vi "Ximea Set ROI.vi"(8 "error in":errorcluster, 9 "Image Ref":T6, 10 "Ximea Camera Cluster":T1, 11 "xiCam In":refnum<k24>) -> (0 "error out":errorcluster, 3 "xiCam Out":refnum<k24>)   [LabVIEW 2016]
uses:
  C:/Users/Ries Lab/Documents/Microscope Control from Sheng Account/Microscope-Control/Device Library/Cameras/Ximea/xiLIB_64bit/xiLIB/xiCamLib/API/x64/xiApi.NETX64.dll
  xiLIB_64bit/xiLIB/xiCamLib/API/x64/xiApi.NETX64.dll
  <vilib>/vision/Image Controls.llb/IMAQ Image.ctl
  Ximea Controls/Ximea Notifier Element.ctl
  Ximea Controls/Ximea Actions.ctl
  Ximea Controls/Ximea Parameters.ctl
  Ximea Controls/Ximea Parameter List.ctl
  Ximea Controls/Ximea ROI.ctl
  Camera Controls/Camera IMAQ Key Info.ctl
  xiLIB_64bit/xiLIB/xiCamLib/xiCam/PRM/PRM/PRM_v2.ctl
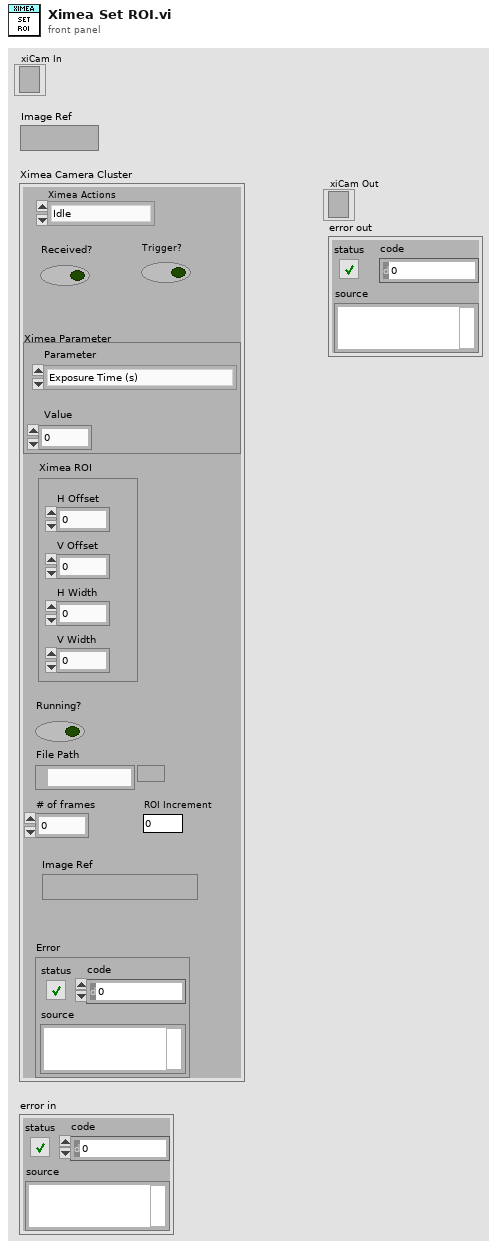
[diagram p1: front panel]
types:
  T1 = typedef "Ximea Notifier Element.ctl" = cluster{"Ximea Actions":T2, "Received?":bool, "Ximea Parameter":T3, "Ximea ROI":T5, "Running?":bool, "File Path":path, "# of frames":u32, "Image Ref":T6, "Error":errorcluster, "Trigger?":bool, "ROI Increment":i32}
  T2 = typedef "Ximea Actions.ctl" = enum16{"Idle", "Error Check", "Preview", "Record", "Soft Trigger", "Abort", "Record Settings", "Set Parameter", "Get Parameter", "Set ROI", "Get ROI", "Status", "Quit"}
  T3 = typedef "Ximea Parameters.ctl" = cluster{"Parameter":T4, "Value":sgl}
  T4 = typedef "Ximea Parameter List.ctl" = enum16{"Exposure Time (s)", "Gain"}
  T5 = typedef "Ximea ROI.ctl" = cluster{"H Offset":i32, "V Offset":i32, "H Width":i32, "V Width":i32}
  T6 = typedef "IMAQ Image.ctl" = refnum<image>
  T7 = typedef "PRM_v2.ctl" = enum16{"ACQ_BUFFER_SIZE", "ACQ_FRAME_BURST_COUNT", "ACQ_TIMING_MODE", "ACQ_TRANSPORT_BUFFER_SIZE", "AE_MAX_LIMIT", "AEAG", "AEAG_LEVEL", "API_VERSION", "AG_MAX_LIMIT", "APPLY_CMS", "AUTO_BANDWIDTH_CALCULATION", "AUTO_WB", "AVAILABLE_BANDWIDTH", "AVAILABLE_BANDWIDTH_MAX", "AVAILABLE_BANDWIDTH_MIN", "BUFFER_POLICY", "BUFFERS_QUEUE_SIZE", "CC_MATRIX_00", "CC_MATRIX_01", "CC_MATRIX_02", "CC_MATRIX_03", "CC_MATRIX_10", "CC_MATRIX_11", "CC_MATRIX_12", "CC_MATRIX_13", "CC_MATRIX_20", "CC_MATRIX_21", "CC_MATRIX_22", "CC_MATRIX_23", "CC_MATRIX_30", "CC_MATRIX_31", "CC_MATRIX_32", "CC_MATRIX_33", "CHIP_TEMP", "CMS", "COLOR_FILTER_ARRAY", "COOLING", "DEBOUNCE_EN", "DEBOUNCE_POL", "DEBOUNCE_T0", "DEBOUNCE_T1", "DEBUG_LEVEL", "DEFAULT_CC_MATRIX", "DEVICE_INSTANCE_PATH", "DEVICE_MODEL_ID", "DEVICE_NAME", "DEVICE_SN", "DEVICE_TYPE", "DEVICE_USER_ID", "DOWNSAMPLING", "DOWNSAMPLING_TYPE", "DRV_VERSION", "EXP_PRIORITY", "EXPOSURE", "EXPOSURE_MAX", "EXPOSURE_MIN", "FFS_FILE_NAME", "FPGA1_VERSION", "FRAMERATE", "FRAMERATE_MAX", "FRAMERATE_MIN", "FREE_FFS_SIZE", "GAIN", "GAIN_MAX", "GAIN_MIN", "GAMMAC", "GAMMAY", "GPI_LEVEL", "GPI_MODE", "GPI_SELECTOR", "GPO_MODE", "GPO_SELECTOR", "HDR", "HDR_T1", "HDR_T2", "HEIGHT", "HEIGHT_MAX", "HEIGHT_MIN", "HOUSE_TEMP", "IMAGE_DATA_FORMAT", "IMAGE_IS_COLOR", "INPUT_CMS_PROFILE", "IS_COOLED", "IS_DEVICE_EXIST", "KNEEPOINT1", "KNEEPOINT2", "LED_MODE", "LED_SELECTOR", "LIMIT_BANDWIDTH", "LIMIT_BANDWIDTH_MAX", "LIMIT_BANDWIDTH_MIN", "LUT_EN", "LUT_INDEX", "LUT_INDEX_MAX", "LUT_INDEX_MIN", "LUT_VALUE", "LUT_VALUE_MAX", "LUT_VALUE_MIN", "MANUAL_WB", "MCU1_VERSION", "MCU2_VERSION", "OFFSET_X", "OFFSET_X_MAX", "OFFSET_X_MIN", "OFFSET_Y", "OFFSET_Y_MAX", "OFFSET_Y_MIN", "OUTPUT_CMS_PROFILE", "OUTPUT_DATA_BIT_DEPTH", "OUTPUT_DATA_PACKING", "READ_FILE_FFS", "RECENT_FRAME", "SENSOR_DATA_BIT_DEPTH", "SENSOR_MODE", "SENSOR_TAPS", "SHARPNESS", "SHUTTER_TYPE", "TARGET_TEMP", "TRG_DELAY", "TRG_SELECTOR", "TRG_SOFTWARE", "TRG_SOURCE", "USED_FFS_SIZE", "WB_KB", "WB_KG", "WB_KR", "WIDTH", "WIDTH_MAX", "WIDTH_MIN", "WRITE_FILE_FFS", "ACQ_BUFFER_SIZE_UNIT", "ACQ_TRANSPORT_BUFFER_COMMIT", "AEAG_ROI_HEIGHT", "AEAG_ROI_OFFSET_X", "AEAG_ROU_OFFSET_Y", "AEAG_ROI_WIDTH", "API_CONTEXT_LIST", "BINNING_HORIZONTAL", "BINNING_SELECTOR", "BINNING_VERTICAL", "COLUMN_FPN_CORRECTION", "COUNTER_SELECTOR", "COUNTER_VALUE", "DECIMATION_HORIZONTAL", "DECIMATION_SELECTOR", "DECIMATION_VERTICAL", "DEVICE_ID", "DEVICE_LOCATION_PATH", "DEVICE_MANIFEST", "DEVICE_RESET", "DEVICE_SENS_SN", "EXPOSURE_BURST_COUNT", "FFS_ACCESS_KEY", "GAIN_SELECTOR", "HW_REVISION", "IMAGE_BLACK_LEVEL", "IMAGE_DATA_BIT_DEPTH", "IMAGE_DATA_FORMAT_RGB32_ALPHA", "IMAGE_PAYLOAD_SIZE", "LENS_APERTURE_VALUE", "LENS_FEATURE", "LENS_FEATURE_SELECTOR", "LENS_FOCAL_LENGTH", "LENS_FOCUS_DISTANCE", "LENS_FOCUS_MOVE", "LENS_FOCUS_MOVEMENT_VALUE", "LENS_MODE", "OUTPUT_DATA_PACKING_TYPE", "SENSOR_CLOCK_FREQ_HZ", "SENSOR_CLOCK_FREQ_INDEX", "SENSOR_FEATURE_SELECTOR", "SENSOR_FEATURE_VALUE", "SENSOR_OUTPUT_CHANNEL_COUNT", "TRANSPORT_PIXEL_FORMAT", "TS_RST_MODE", "TS_RST_SOURCE", "SENS_DEFECTS_CORR_LIST_SELECTOR", "SENS_DEFECTS_CORR", "SENS_DEFECTS_CORR_LIST_CONTENT", "DEVICE_UNIT_SELECTOR", "DEVICE_UNIT_REGISTER_SELECTOR", "DEVICE_UNIT_REGISTER_VALUE"}
  T8 = typedef "Camera IMAQ Key Info.ctl" = cluster{"Frame":u32, "Sensor Height":i32, "Sensor Width":i32, "ROI Height":i32, "ROI Width":i32, "ROI Enable?":bool, "Bit per Pixel":u8}
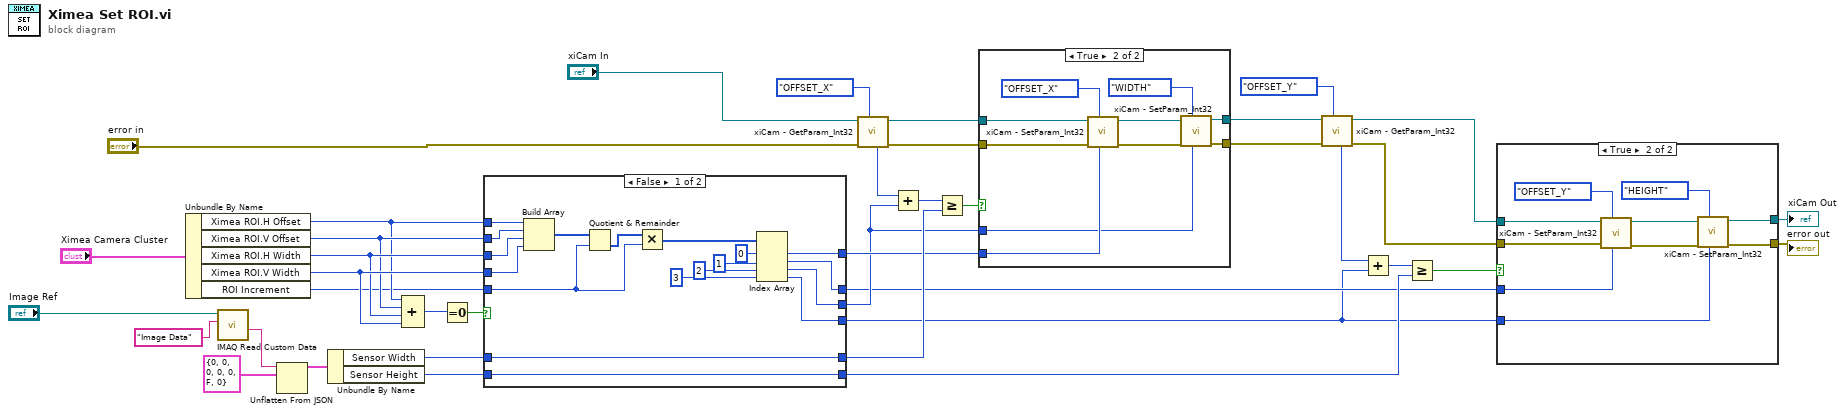
[diagram p0: block diagram]
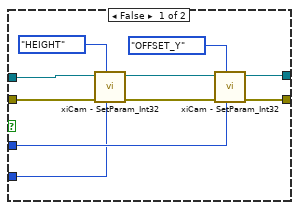
[diagram p2: hidden frame]
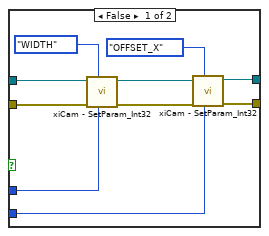
[diagram p3: hidden frame]
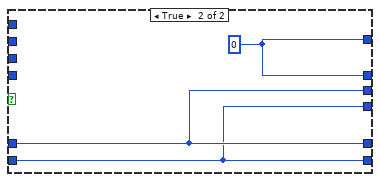
[diagram p4: hidden frame]
diagram:
  n1 = Unbundle By Name("Ximea Camera Cluster") -> ("Ximea ROI.H Offset"=w28:i32, "Ximea ROI.V Offset"=w29:i32, "Ximea ROI.H Width"=w30:i32, "Ximea ROI.V Width"=w31:i32, "ROI Increment"=w27:i32)
  n2 = call "IMAQ Read Custom Data"("Key"="Image Data", "Image"="Image Ref") -> ("Custom Data Out"=w21:string)  [unwired: 7 in, 2 out]
  n3 = Unflatten From JSON(JSON string=w21, type and defaults=T8 {"Frame"=0, "Sensor Height"=0, "Sensor Width"=0, "ROI Height"=0, "ROI Width"=0, "ROI Enable?"=FALSE, "Bit per Pixel"=0} ("Camera IMAQ Key Info")) -> (value=w22:T8)  [unwired: 5 in, 1 out]
  n4 = Unbundle By Name(w22) -> ("Sensor Width"=w25:i32, "Sensor Height"=w26:i32)
  n5 = Compound Arithmetic op=ADD(w28, w29, w30, w31) -> (w19:i32)
  n6 = Equal To 0?(x=w19) -> (x = 0?=w24:bool)
  n7 = case shown="False" w24 {
    tunnel: w25 -> [w41 w59]
    tunnel: w26 -> [w40 w58]
    tunnel: [w44 w59] -> w14
    tunnel: [w43 w58] -> w3
    tunnel: w27 -> [w48 _]
    tunnel: w28 -> [w57 _]
    tunnel: w29 -> [w56 _]
    tunnel: w30 -> [w55 _]
    tunnel: w31 -> [w54 _]
    tunnel: [w46 w60] -> w15
    tunnel: [w45 w60] -> w4
    tunnel: [w41 w59] -> w38
    tunnel: [w40 w58] -> w9
    frame False {
      n8 = Build Array(w57, w56, w55, w54) -> (w53:i32[])
      n9 = Quotient & Remainder(x=w53, y=w48) -> (floor(x/y)=w42:i32[])  [unwired: 1 out]
      n10 = Multiply(x=w42, y=w48) -> (x*y=w47:i32[])
      n11 = Index Array(array=w47, index #1=0 ("index"), index #2=1 ("index"), index #3=2 ("index"), index #4=3 ("index")) -> (element #1=w46:i32, element #2=w45:i32, element #3=w44:i32, element #4=w43:i32)
    }
    frame True {
      w60 = 0
    }
  }
  n12 = call "xiCam - GetParam_Int32.vi"("PRM"=PRM_v2."OFFSET_X", "error in (no error)"="error in", "xiCam In"="xiCam In") -> ("error out"=w16:errorcluster, "xiCam Out"=w17:refnum<k24>, "Int32_Value"=w36:i32)  [unwired: 6 in]
  n13 = Add(x=w36, y=w14) -> (x+y=w37:i32)
  n14 = Greater Or Equal?(x=w37, y=w38) -> (x >= y?=w39:bool)
  n15 = case shown="True" w39 {
    tunnel: w17 -> [w66 w79]
    tunnel: w16 -> [w65 w75]
    tunnel: w15 -> [w64 w78]
    tunnel: w14 -> [w63 w73]
    tunnel: [w62 w72] -> w12
    tunnel: [w61 w71] -> w11
    frame False {
      n16 = call "xiCam - SetParam_Int32.vi"("Int32_Value"=w63, "PRM"=PRM_v2."WIDTH", "error in (no error)"=w65, "xiCam In"=w66) -> ("error out"=w70:errorcluster, "xiCam Out"=w69:refnum<k24>)  [unwired: 6 in]
      n17 = call "xiCam - SetParam_Int32.vi"("Int32_Value"=w64, "PRM"=PRM_v2."OFFSET_X", "error in (no error)"=w70, "xiCam In"=w69) -> ("error out"=w61:errorcluster, "xiCam Out"=w62:refnum<k24>)  [unwired: 6 in]
    }
    frame True {
      n18 = call "xiCam - SetParam_Int32.vi"("Int32_Value"=w78, "PRM"=PRM_v2."OFFSET_X", "error in (no error)"=w75, "xiCam In"=w79) -> ("error out"=w74:errorcluster, "xiCam Out"=w76:refnum<k24>)  [unwired: 6 in]
      n19 = call "xiCam - SetParam_Int32.vi"("Int32_Value"=w73, "PRM"=PRM_v2."WIDTH", "error in (no error)"=w74, "xiCam In"=w76) -> ("error out"=w71:errorcluster, "xiCam Out"=w72:refnum<k24>)  [unwired: 6 in]
    }
  }
  n20 = call "xiCam - GetParam_Int32.vi"("PRM"=PRM_v2."OFFSET_Y", "error in (no error)"=w11, "xiCam In"=w12) -> ("error out"=w6:errorcluster, "xiCam Out"=w7:refnum<k24>, "Int32_Value"=w5:i32)  [unwired: 6 in]
  n21 = Add(x=w5, y=w3) -> (x+y=w10:i32)
  n22 = Greater Or Equal?(x=w10, y=w9) -> (x >= y?=w8:bool)
  n23 = case shown="True" w8 {
    tunnel: w7 -> [w89 w99]
    tunnel: w6 -> [w88 w98]
    tunnel: w4 -> [w84 w94]
    tunnel: w3 -> [w83 w93]
    tunnel: [w82 w92] -> w2
    tunnel: [w81 w91] -> w1
    frame False {
      n24 = call "xiCam - SetParam_Int32.vi"("Int32_Value"=w83, "PRM"=PRM_v2."HEIGHT", "error in (no error)"=w88, "xiCam In"=w89) -> ("error out"=w85:errorcluster, "xiCam Out"=w86:refnum<k24>)  [unwired: 6 in]
      n25 = call "xiCam - SetParam_Int32.vi"("Int32_Value"=w84, "PRM"=PRM_v2."OFFSET_Y", "error in (no error)"=w85, "xiCam In"=w86) -> ("error out"=w81:errorcluster, "xiCam Out"=w82:refnum<k24>)  [unwired: 6 in]
    }
    frame True {
      n26 = call "xiCam - SetParam_Int32.vi"("Int32_Value"=w94, "PRM"=PRM_v2."OFFSET_Y", "error in (no error)"=w98, "xiCam In"=w99) -> ("error out"=w95:errorcluster, "xiCam Out"=w96:refnum<k24>)  [unwired: 6 in]
      n27 = call "xiCam - SetParam_Int32.vi"("Int32_Value"=w93, "PRM"=PRM_v2."HEIGHT", "error in (no error)"=w95, "xiCam In"=w96) -> ("error out"=w91:errorcluster, "xiCam Out"=w92:refnum<k24>)  [unwired: 6 in]
    }
  }
  "xiCam Out" <- w2
  "error out" <- w1
